vi "lsl push chunk buf.vi"(7 "data_elements":u32, 8 "error in (no error)":errorcluster, 9 "lengths":u32, 10 "data":string, 11 "out":cluster{}) -> (0 "error out":errorcluster, 2 "function return":i32, 3 "out out":cluster{})   [LabVIEW 2016, in "Lab Streaming Layer.lvlib"]
doc: "extern LIBLSL_C_API int32_t lsl_push_chunk_buf(lsl_outlet out, const char **data, const uint32_t*lengths, unsigned long data_elements);"
uses:
  Lab Streaming Layer.lvlib
  liblsl-LabVIEW-master/liblsl-LabVIEW-master/lsl.dll
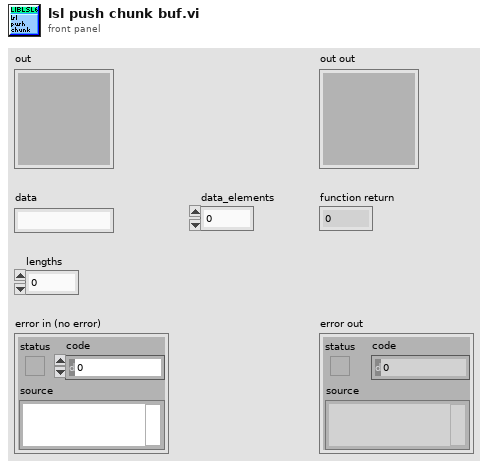
[diagram p1: front panel]
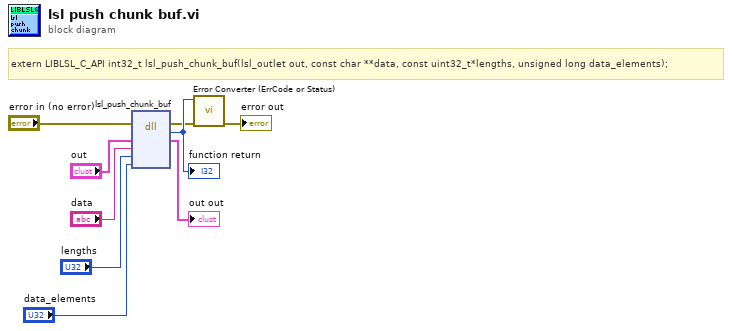
[diagram p0: block diagram]
diagram:
  # "extern LIBLSL_C_API int32_t lsl_push_chunk_buf(lsl_outlet out, const char **data, const uint32_t*lengths, unsigned long data_elements);"
  n1 = dll-call lib="E:/LabStreamingLayer/liblsl-LabVIEW-master/liblsl-LabVIEW-master/lsl.dll" fn="lsl_push_chunk_buf"(error in="error in (no error)", "out"="out", "data"="data", "lengths"="lengths", "data_elements"="data_elements") -> (error out=w2:errorcluster, "return type"=w9:i32, "out"=→"out out":cluster{})  [unwired: 5 in, 1 out]
  "function return" <- w9
  n2 = call "Error Converter (ErrCode or Status).vi"("error in (no error)"=w2, "error code"=w9) -> ("error out"=→"error out":errorcluster)  [unwired: 9 in]
